vi "Low Pass Filter.vi"() -> ()   [LabVIEW 2013]
panel:
  out "Waveform Graph 2":dynamicdata(graph)
  out "Waveform Graph":dynamicdata(graph)
  in  "Numeric":dbl
  in  "stop":bool
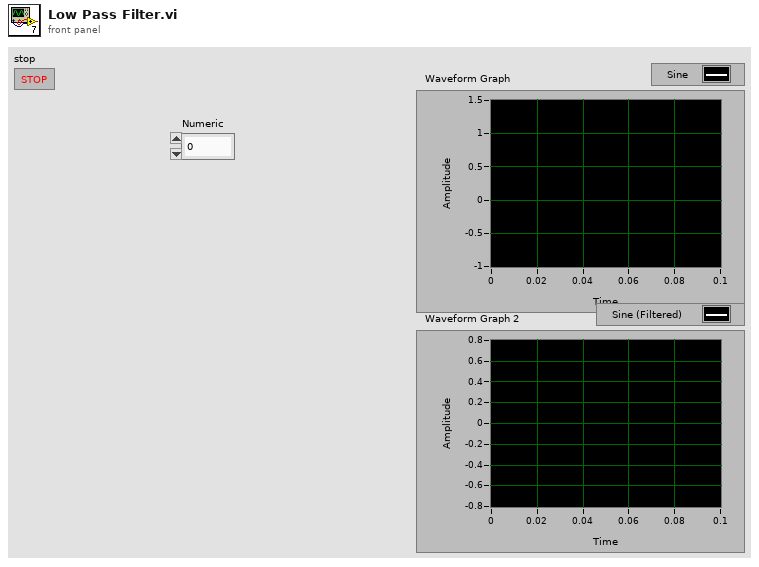
[diagram p1: front panel]
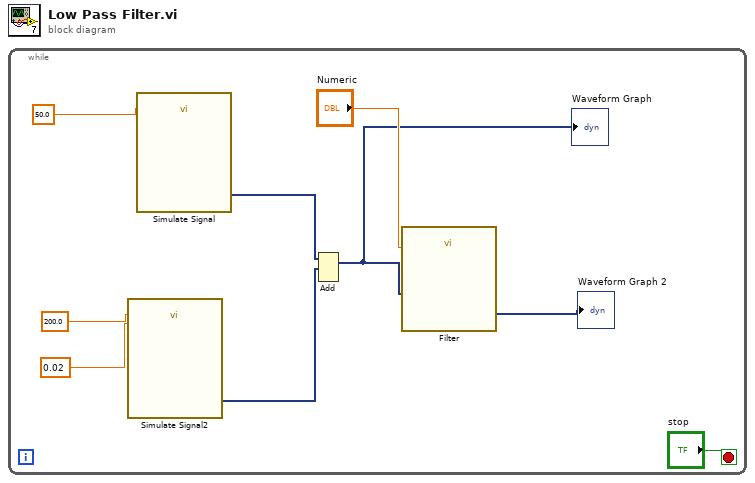
[diagram p0: block diagram]
diagram:
  n1 = while {
    stop <- "stop" stop-if-true
    n2 = call "Simulate Signal2"("Frequency"=200.0, "Amplitude"=0.02) -> ("Sine"=w4:dynamicdata)  [unwired: 12 in, 1 out]
    n3 = call "Simulate Signal"("Frequency"=50.0) -> ("Sine"=w5:dynamicdata)  [unwired: 13 in, 1 out]
    n4 = Add(1:w4, 2:w5) -> (0:w2:dynamicdata)  [unwired: 1 in, 1 out]
    "Waveform Graph" <- w2
    n5 = call "Filter"("Lower Cut-Off"="Numeric", "Signal"=w2) -> ("Filtered Signal"=→"Waveform Graph 2":dynamicdata)  [unwired: 8 in, 1 out]
  }
